vi "Display Window.vi"(0 "Py Doc in":refnum<class "Py Doc.lvclass">, 11 "error in (no error)":errorcluster) -> (4 "Py Doc out":refnum<class "Py Doc.lvclass">, 15 "error out":errorcluster)   [LabVIEW 2016, in "Py Doc.lvclass"]
uses:
  Py Doc.lvclass
  C:/Users/namratha.balakrishna/Desktop/source code/MDI/D/MDI Project/source code/Document/Document.lvclass
  Document.lvclass/Document.ctl
  Py Doc.lvclass/Py Doc.ctl
  user32.dll
  Document.lvclass
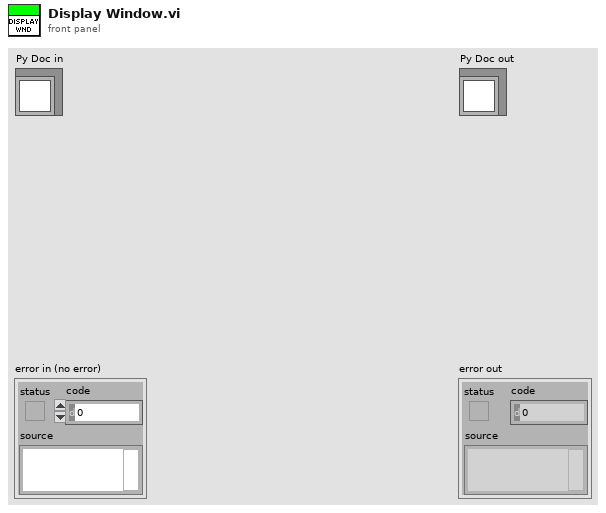
[diagram p1: front panel]
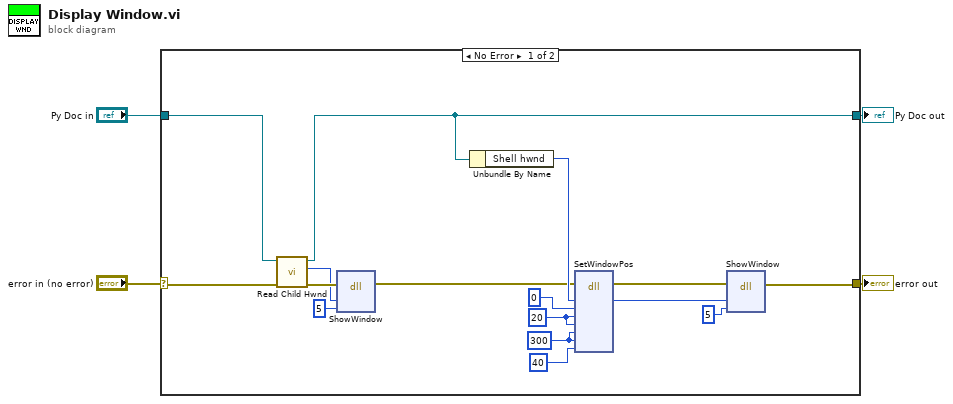
[diagram p0: block diagram]
diagram:
  n1 = case shown="No Error" "error in (no error)" {
    selector: "error in (no error)" -> [w8 w22]
    tunnel: [w12 w22] -> w3
    tunnel: [w5 w21] -> w1
    tunnel: "Py Doc in" -> [w6 w21]
    frame No Error {
      w16 = 300 ("cx")
      w17 = 20 ("x")
      n2 = call "Read Child Hwnd.vi"("error in (no error)"=w8, "Document in"=w6) -> ("error out"=w10:errorcluster, "Child Hwnd"=w9:u32, "Document out"=w5:refnum<class "Py Doc.lvclass">)  [unwired: 7 in]
      n3 = dll-call lib="user32.dll" fn="ShowWindow"(error in=w10, "hwnd"=w9, "nCmdShow"=u32 5) -> (error out=w7:errorcluster)  [unwired: 5 in, 1 out]
      n4 = Unbundle By Name(w5) -> ("Shell hwnd"=w15:u32)
      n5 = dll-call lib="user32.dll" fn="SetWindowPos"(error in=w7, "Hwnd"=w15, "hwndInsertafter"=0, "x"=w17, "y"=w17, "cx"=w16, "cy"=w16, "uflags"=40) -> (error out=w14:errorcluster, "Hwnd"=w13:u32)  [unwired: 9 in, 1 out]
      n6 = dll-call lib="user32.dll" fn="ShowWindow"(error in=w14, "hwnd"=w13, "nCmdShow"=u32 5) -> (error out=w12:errorcluster)  [unwired: 5 in, 1 out]
    }
    frame Error {
    }
  }
  "error out" <- w3
  "Py Doc out" <- w1
